vi "QMH Add Message to Queue.vi"   [LabVIEW 2011]
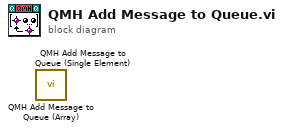
[diagram p0: block diagram]
diagram:
  n1 = call "QMH Add Message to Queue (Array).vi"() -> ()  [unwired: 10 in, 2 out]
  n2 = call "QMH Add Message to Queue (Single Element).vi"() -> ()  [unwired: 10 in, 2 out]
